vi "test Add-Read Terminals and Acyclic Frames.vi"(8 "error in":errorcluster, 11 "TestCase in":refnum<class "Scripting.lvclass">) -> (0 "error out":errorcluster, 3 "TestCase out":refnum<class "Scripting.lvclass">)   [LabVIEW 2020, in "Scripting.lvclass"]
uses:
  Scripting.lvclass
  C:/dev/git/niveristand-custom-device-testing-tools/VeriStandScriptingTestCase/VeriStandScriptingTestCase.lvclass
  Shared/Address.ctl
  niveristand-custom-device-testing-tools/VeriStandScriptingTestCase/VeriStandScriptingTestCase.lvclass/VeriStandScriptingTestCase.ctl
  niveristand-custom-device-testing-tools/VeriStandScriptingTestCase/Read Target.vi
  NationalInstruments.VeriStand.SystemDefinitionAPI
  Scripting/AIM MIL-STD-1553 Scripting.lvlib
  <vilib>/addons/_JKI Toolkits/VI Tester/TestCase.llb/TestCase.lvclass
  C:/Program Files (x86)/National Instruments/LabVIEW 2020/vi.lib/addons/_JKI Toolkits/VI Tester/TestCase.llb/TestCase.lvclass
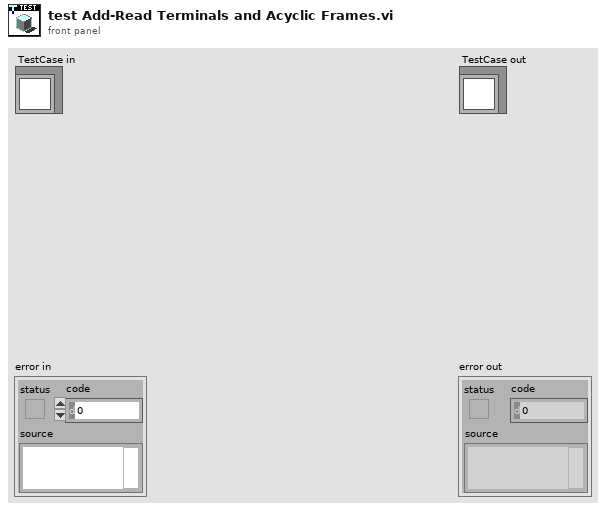
[diagram p1: front panel]
types:
  T1 = typedef "Address.ctl" = u16
  T2 = typedef "Custom Device API.lvlib/Custom Device Item Ref.ctl" = u64
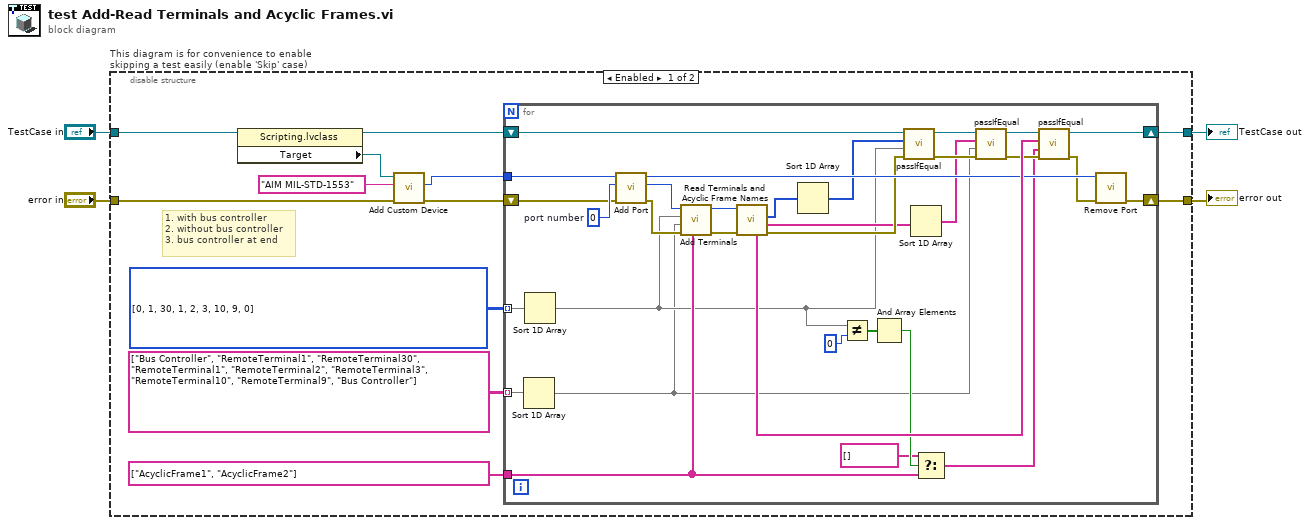
[diagram p0: block diagram]
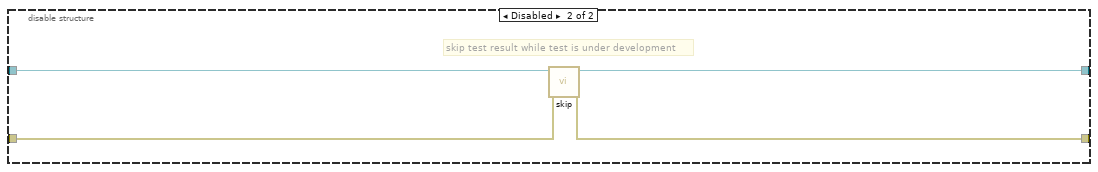
[diagram p2: hidden frame]
diagram:
  n1 = disable-structure "This diagram is for convenience to enable skipping a test easily (enable 'Skip' case)" shown="Enabled" {
    disable-tunnel: "TestCase in" -> [w14 w52]
    disable-tunnel: [w9 w50] -> w4
    disable-tunnel: [w5 w51] -> w2
    disable-tunnel: "error in" -> [w16 w49]
    frame Enabled {
      # "1. with bus controller\n2. without bus controller\n3. bus controller at end"
      n2 = property class="Scripting.lvclass"(reference=w14) -> (reference out=w12:refnum<class "Scripting.lvclass">, "Target"=w13:refnum<k24>)  [unwired: 1 in, 1 out]
      n3 = call "Add Custom Device.vi"("error in"=w16, "custom device name"="AIM MIL-STD-1553" ("name"), "target"=w13) -> ("error out"=w11:errorcluster, "custom device"=w10:T2)  [unwired: 6 in, 1 out]
      n4 = for {
        tunnel: w10 -> [w45]
        tunnel: string[] ["AcyclicFrame1", "AcyclicFrame2"] ("acyclic frame names") -> [w27]
        tunnel: T1[][] [[0, 1, 30], [1, 2, 3], [10, 9, 0]] ("terminal addresses") -> [w24] mode=indexing
        tunnel: string[][] [["Bus Controller", "RemoteTerminal1", "RemoteTerminal30"], ["RemoteTerminal1", "RemoteTerminal2", "RemoteTerminal3"], ["RemoteTerminal10", "RemoteTerminal9", "Bus Controller"]] ("terminal names") -> [w18] mode=indexing
        shift-right: [w38] -> w9
        shift-left: w12 -> [w48]
        shift-right: [w31] -> w5
        shift-left: w11 -> [w46]
        w47 = 0  # port number
        n5 = Sort 1D Array(array=w18) -> (sorted array=w17:string[])
        n6 = Sort 1D Array(array=w24) -> (sorted array=w19:T1[])
        n7 = call "Add Port.vi"("error in"=w46, "port number"=w47, "custom device"=w45) -> ("error out"=w43:errorcluster, "port"=w44:T2, "custom device out"=w36:T2)  [unwired: 6 in]
        n8 = call "Add Terminals.vi"("acyclic frame names"=w27, "error in"=w43, "terminal names"=w17, "terminal addresses"=w19, "port"=w44) -> ("error out"=w41:errorcluster, "port out"=w42:T2)  [unwired: 5 in]
        n9 = call "Read Terminals and Acyclic Frame Names.vi"("error in"=w41, "port"=w42) -> ("error out"=w35:errorcluster, "terminal names"=w21:string[], "terminals"=w23:T1[], "acyclic frame names"=w37:string[])  [unwired: 5 in, 1 out]
        n10 = Sort 1D Array(array=w23) -> (sorted array=w22:T1[])
        n11 = Not Equal?(x=w19, y=0) -> (x != y?=w29:bool[])
        n12 = And Array Elements(Boolean array=w29) -> (logical AND=w28:bool)
        n13 = call-dynamic "passIfEqual.vi"("error in (no error)"=w35, "y"=w19, "x"=w22, "TestCase in"=w48) -> ("error out"=w34:errorcluster, "TestCase out"=w40:refnum<class "Scripting.lvclass">)  [unwired: 6 in]
        n14 = Sort 1D Array(array=w21) -> (sorted array=w20:string[])
        n15 = Select(t=string[] [] ("acyclic frame names"), s=w28, f=w27) -> (s? t:f=w25:string[])
        n16 = call-dynamic "passIfEqual.vi"("error in (no error)"=w34, "y"=w17, "x"=w20, "TestCase in"=w40) -> ("error out"=w33:errorcluster, "TestCase out"=w39:refnum<class "Scripting.lvclass">)  [unwired: 6 in]
        n17 = call-dynamic "passIfEqual.vi"("error in (no error)"=w33, "y"=w25, "x"=w37, "TestCase in"=w39) -> ("error out"=w32:errorcluster, "TestCase out"=w38:refnum<class "Scripting.lvclass">)  [unwired: 6 in]
        n18 = call "Remove Port.vi"("error in"=w32, "custom device ref"=w36) -> ("error out"=w31:errorcluster)  [unwired: 7 in, 2 out]
      }
    }
    frame Disabled {
      # "skip test result while test is under development"
      n19 = call <vilib>:"skip.vi"("error in (no error)"=w49, "TestCase in"=w52) -> ("error out"=w51:errorcluster, "TestCase out"=w50:refnum<class "Scripting.lvclass">)  [unwired: 8 in]
    }
  }
  "error out" <- w2
  "TestCase out" <- w4
